vi "Target.vi"() -> ()   [LabVIEW 2017]
uses:
  shared/Kobuki Sensor Display.ctl
  controls/StatesEnum.ctl
  <vilib>/Platform/TimedLoop/XDataNode/timing_clust.ctl
  <vilib>/Platform/TimedLoop/XDataNode/nitl_modes.ctl
  <vilib>/Platform/TimedLoop/XDataNode/wakeup.ctl
  <vilib>/myRIO/Instrument Drivers/Onboard IO/UART/typedef/VISA Configuration.ctl
  shared/Sensors.ctl
  shared/Accelerometer.ctl
  Kobuki/KobukiSensors.ctl
  Kobuki/Kobuki Bumps and WheelDrops.ctl
  Kobuki/Kobuki Buttons.ctl
  <vilib>/myRIO/Common/Instrument Driver Framework/myRIO v1.0/UART/vis/myRIO v1.0 Close UART.vi
  <vilib>/myRIO/Common/Instrument Driver Framework/myRIO v1.0/myRIO v1.1 Open.vi
  Global Light Sensor.vi
  <vilib>/Instr/_visa.llb/VISA Configure Serial Port (Instr).vi
  <vilib>/myRIO/Common/Instrument Driver Framework/Utilities/vis/FPGA Ref Manager.vi
  <vilib>/myRIO/Common/Instrument Driver Framework/myRIO v1.0/myRIO v1.0 Reset FPGA.vi
  <vilib>/myRIO/Common/Instrument Driver Framework/myRIO v1.0/IRQ/vis/myRIO v1.0 IRQ Info FGV.vi
  <vilib>/myRIO/Common/Instrument Driver Framework/myRIO v1.0/IRQ/vis/myRIO v1.0 Timer IRQ Info FGV.vi
  <vilib>/myRIO/Common/Instrument Driver Framework/myRIO v1.0/IRQ/vis/myRIO v1.0 ISR Agent.vi
  <vilib>/Platform/TimedLoop/XDataNode/XDataNode.xnode
  <vilib>/myRIO/Express VI/Onboard IO/UART/UART Express VI.xnode
  <vilib>/myRIO/Instrument Drivers/Utilities/Utilities.lvlib
  <vilib>/Platform/TimedLoop/XDataNode/XDNodeRunTimeDep.lvlib
  <vilib>/myRIO/Instrument Drivers/Onboard IO/UART/UART.lvlib
panel:
  in  "Pause":bool
  in  "Tab Control":T1(tab)
  out "Kobuki Sensors (graphical)":T2 {"Right Wheel (mm/s)" scale=-500.0..500.0; "Left Wheel (mm/s)" scale=-500.0..500.0}
  out "Charge Status":i8(ring) items=["DISCHARGING"=0, "DOCKING_CHARGED"=2, "DOCKING_CHARGING"=6, "ADAPTER_CHARGED"=18, "ADAPTER_CHARGING"=22]
  out "Kobuki Battery Voltage":dbl(knob)=12000.0 scale=12.0..16.4 scale format="%#.1f"
  out "CurrentState":T4
  out "Loop Duration":i64
  out "error out":errorcluster
  in  "stop":bool
  out "Target Running":bool
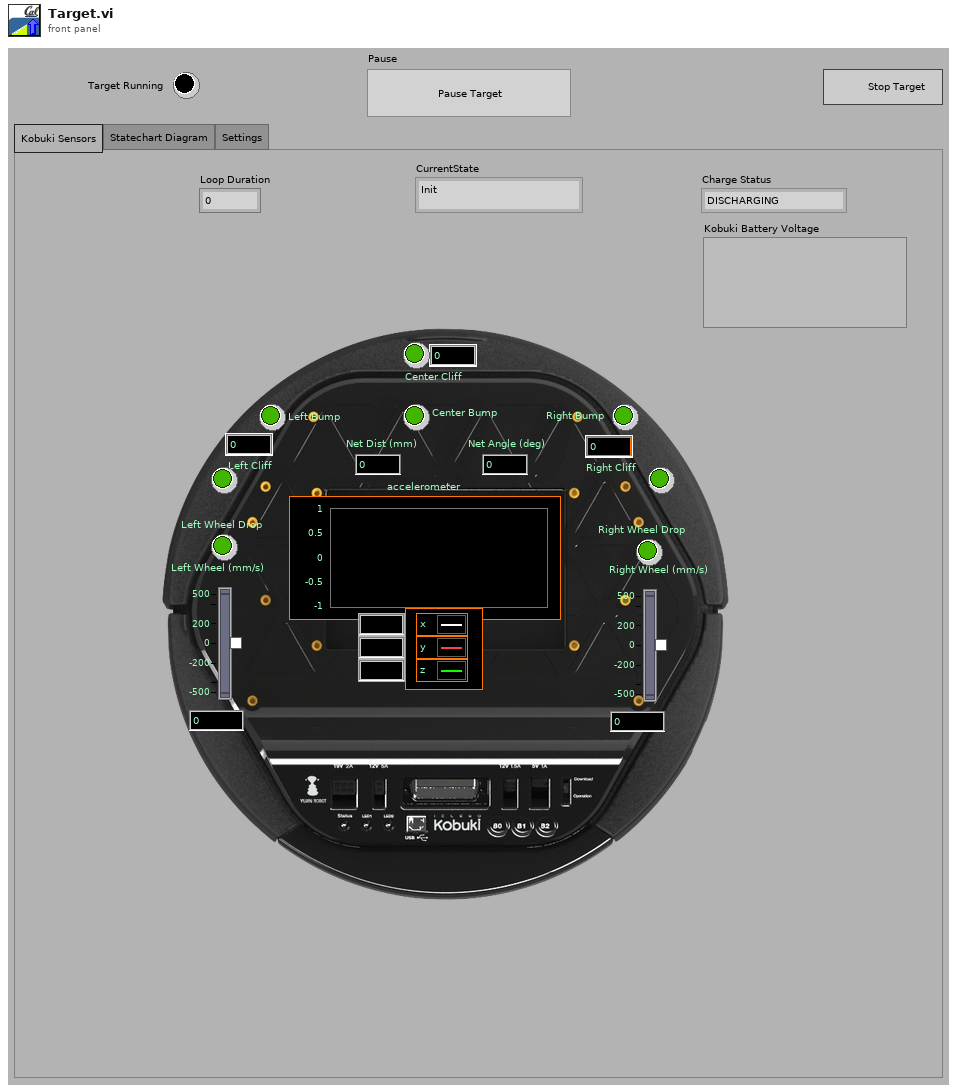
[diagram p1: front panel]
types:
  T1 = enum32{"Kobuki Sensors", "Statechart Diagram", "Settings"}
  T2 = typedef "Kobuki Sensor Display.ctl" = cluster{"Center Bump":bool, "Left Wheel Drop":bool, "Right Wheel Drop":bool, "Left Bump":bool, "Right Bump":bool, "Left Cliff":bool, "Center Cliff":bool, "Right Cliff":bool, "Net Dist (mm)":i32, "Net Angle (deg)":i32, "Left Cliff":u16, "Center Cliff":u16, "Right Cliff":u16, "  Left Wheel (mm/s)":i16, "Right Wheel (mm/s)":i16, "accelerometer":T3}
  T3 = typedef "Accelerometer.ctl" = cluster{"x axis (g)":dbl, "y axis (g)":dbl, "z axis (g)":dbl}
  T4 = typedef "StatesEnum.ctl" = enum16{"Init", "Center Cliff\n", "Pause", "Drive", "U.Turn", "L.Cliff", "R.Cliff", "Shut", "L.Bump", "R.Bump", "Red Light"}
  T5 = typedef "XDNodeRunTimeDep.lvlib/timing_clust.ctl" = cluster{"Expected End [f-1]":u64, "Actual End [f-1]":u64, "Finished Late? [f-1]":bool, "Expected End [i-1]":u64, "Actual End [i-1]":u64, "Finished Late? [i-1]":bool, "Expected Start [i]":u64, "Actual Start [i]":u64, "Expected Start [f]":u64, "Actual Start [f]":u64, "Source Name":string, "Structure Name":string, "Period":i64, "Deadline":i64, "Offset":i64, "Start":i64, "Priority":i32, "Timeout":i32, "Mode":T6, "Wakeup Reason":T7, "Error":errorcluster, "Source Type":string, "Secondary Source Type":string, "Global End Time":u64, "Global Start Time":u64, "Frame Duration":u64, "Iteration Duration":u64, "Assigned CPU":i32, "I/O Scan Engine Mode":u32}
  T6 = typedef "XDNodeRunTimeDep.lvlib/nitl_modes.ctl" = enum32{"No Change", "Process missed periods, maintain original phase", "Discard missed periods, maintain original phase", "Process missed periods, ignore original phase", "Discard missed periods, ignore original phase"}
  T7 = typedef "XDNodeRunTimeDep.lvlib/wakeup.ctl" = enum32{"Normal", "Aborted", "Asynchronous wakeup", "Timing source error", "Timed loop error", "Timeout"}
  T8 = typedef "Sensors.ctl" = cluster{"net distance (mm)":i32, "net angle (deg)":i32, "accelerometer":T3, "Is Simulator?":bool, "Kobuki Sensors":T9, "Requested Left Wheel Velocity(mm/s)":i32, "Requested Right Wheel Velocity(mm/s)":i32, "Green Light Sensed":bool, "Red Light Sensed":bool}
  T9 = typedef "KobukiSensors.ctl" = cluster{"Bumps + Wheel Drops":T10, "Cliff Left":bool, "Cliff Center":bool, "Cliff Right":bool, "Cliff Left Signal":u16, "Cliff Center Signal":u16, "Cliff Right Signal":u16, "Buttons":T11, "Left Wheel Encoder (ticks)":u16, "Right Wheel Encoder (ticks) ":u16, "Left  Wheel PWM":i8, "Right Wheel PWM":i8, "Left Wheel OverCurrent":bool, "Right Wheel OverCurrent ":bool, "Right Wheel Current (x10mA)":i16, "Left  Wheel Current  (x10mA)":i16, "TimeStamp":u16, "Battery Voltage":dbl, "Angle( of 100deg)":i16, "Angle Rate( of 100 deg/sec)":i16, "Charger Source ":i8}
  T10 = typedef "Kobuki Bumps and WheelDrops.ctl" = cluster{"Wheeldrop Left":bool, "Wheeldrop Right":bool, "Bump Left":bool, "Bump Center":bool, "Bump Right":bool}
  T11 = typedef "Kobuki Buttons.ctl" = cluster{"B0":bool, "B1":bool, "B2":bool}
  T12 = typedef "Outputs.ctl" = cluster{"Left Wheel Speed (mm/s)":i16, "Right Wheel Speed (mm/s)":i16}
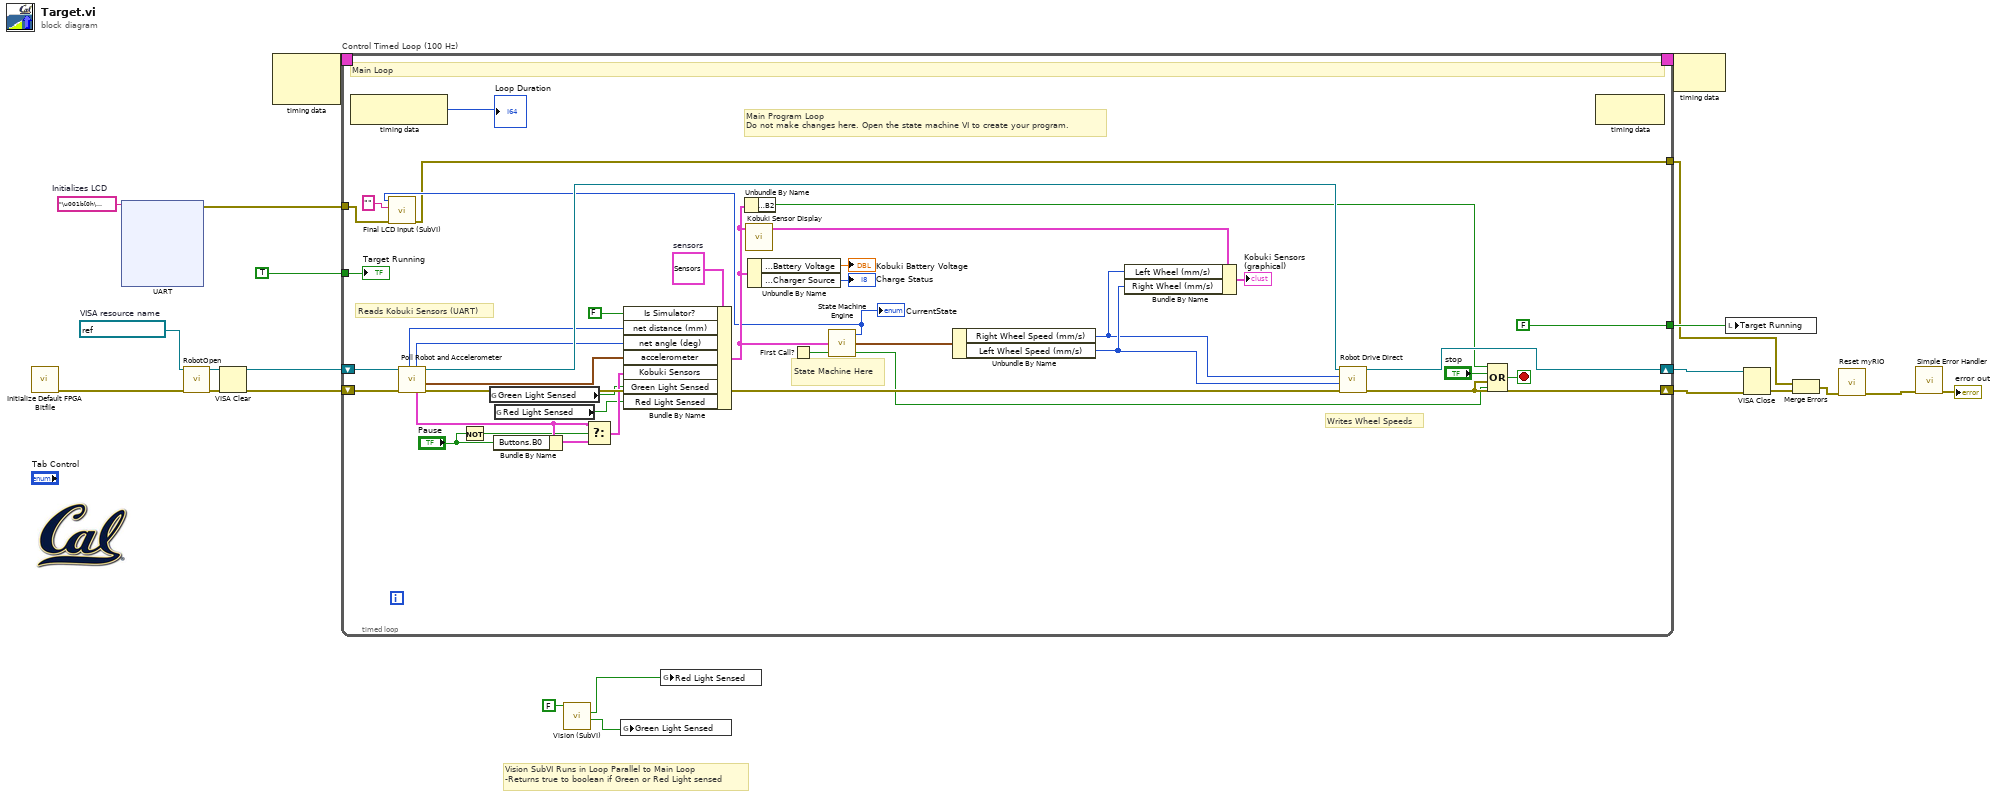
[diagram p0: block diagram]
diagram:
  w7 = "\u001b[0h\u001b[j"  # Initializes LCD
  w19 = refnum<visa-resource-name> "ASRL3::INSTR"  # VISA resource name
  # "Vision SubVI Runs in Loop Parallel to Main Loop\n-Returns true to boolean if Green or Red Light sensed"
  n1 = call <vilib>:"Initialize Default FPGA Bitfile.vi"() -> ("error out"=w17:errorcluster)  [unwired: 11 in]
  n2 = xnode "UART"("Characters to Write"=w7) -> ("error out"=w8:errorcluster)  [unwired: 1 in, 1 out]
  n3 = call "RobotOpen.vi"("error in (no error)"=w17, "Robot Communication port name"=w19) -> ("error out"=w15:errorcluster, "Robot Communication port name out"=w22:refnum<visa-resource-name>)  [unwired: 8 in]
  n4 = VISA Clear(VISA resource name=w22, error in (no error)=w15) -> (VISA resource name out=w13:refnum<visa-resource-name>, error out=w14:errorcluster)
  n5 = node-c288() -> (w10:T5)  [unwired: 2 in]
  n6 = timed-loop "Control Timed Loop (100 Hz)" {
    shift-right: [w60] -> w11
    shift-left: w13 -> [w57]
    shift-right: [w45] -> w12
    shift-left: w14 -> [w56]
    tunnel: TRUE ("stop") -> [w51]
    tunnel: [FALSE ("stop")] -> w20
    timing: w10 -> [_]
    timing-out: [_] -> w9
    tunnel: w8 -> [w28]
    tunnel: [w25] -> w5
    stop <- w59 stop-if-true
    w46 = T8 {"net distance (mm)"=0, "net angle (deg)"=0, "accelerometer"={"x axis (g)"=0.0, "y axis (g)"=0.0, "z axis (g)"=0.0}, "Is Simulator?"=FALSE, "Kobuki Sensors"={"Bumps + Wheel Drops"={"Wheeldrop Left"=FALSE, "Wheeldrop Right"=FALSE, "Bump Left"=FALSE, "Bump Center"=FALSE, "Bump Right"=FALSE}, "Cliff Left"=FALSE, "Cliff Center"=FALSE, "Cliff Right"=FALSE, "Cliff Left Signal"=0, "Cliff Center Signal"=0, "Cliff Right Signal"=0, "Buttons"={"B0"=FALSE, "B1"=FALSE, "B2"=FALSE}, "Left Wheel Encoder (ticks)"=0, "Right Wheel Encoder (ticks) "=0, "Left  Wheel PWM"=0, "Right Wheel PWM"=0, "Left Wheel OverCurrent"=FALSE, "Right Wheel OverCurrent "=FALSE, "Right Wheel Current (x10mA)"=0, "Left  Wheel Current  (x10mA)"=0, "TimeStamp"=0, "Battery Voltage"=0.0, "Angle( of 100deg)"=0, "Angle Rate( of 100 deg/sec)"=0, "Charger Source "=0}, "Requested Left Wheel Velocity(mm/s)"=0, "Requested Right Wheel Velocity(mm/s)"=0, "Green Light Sensed"=FALSE, "Red Light Sensed"=FALSE}  # sensors
    # "Main Program Loop\nDo not make changes here. Open the state machine VI to create your program."
    # "Writes Wheel Speeds"
    # "Reads Kobuki Sensors (UART)"
    # "State Machine Here"
    # "Main Loop"
    n7 = node-c288() -> (→"Loop Duration":i64)  [unwired: 1 in]
    n8 = call "Poll Robot and Accelerometer.vi"("error in"=w56, "UART in"=w57) -> ("error out"=w55:errorcluster, "Acceleration (g)"=w48:T3, "UART out"=w54:refnum<visa-resource-name>, "Kobuki Sensors  out"=w32:T9, "net angle (deg)"=w52:i32, "net distance (mm)"=w53:i32)  [unwired: 4 in]
    n9 = Not(x="Pause") -> (.not. x?=w29:bool)
    n10 = global read "Global Light Sensor.vi" "Green Light Sensed"() -> (w24:bool)
    n11 = Bundle By Name(cluster=w32, "Buttons.B0"="Pause") -> (w33:T9)
    n12 = global read "Global Light Sensor.vi" "Red Light Sensed"() -> (w23:bool)
    n13 = Select(t=w32, s=w29, f=w33) -> (s? t:f=w31:T9)
    n14 = Bundle By Name(cluster=w46, "Is Simulator?"=FALSE, "net distance (mm)"=w53, "net angle (deg)"=w52, "accelerometer"=w48, "Kobuki Sensors"=w31, "Green Light Sensed"=w24, "Red Light Sensed"=w23) -> (w38:T8)
    n15 = Unbundle By Name(w38) -> ("Kobuki Sensors.Buttons.B2"=w49:bool)
    n16 = call "Kobuki Sensor Display.vi"("sensors"=w38) -> ("Kobuki Sensors Display"=w35:T2)  [unwired: 4 in]
    n17 = Unbundle By Name(w38) -> ("Kobuki Sensors.Battery Voltage"=→"Kobuki Battery Voltage":dbl, "Kobuki Sensors.Charger Source"=→"Charge Status":i8)
    n18 = First Call?() -> (First Call?: T/F=w40:bool)
    n19 = call "State Machine Engine.vi"("Init?"=w40, "Inputs"=w38) -> ("Terminated?"=w39:bool, "Outputs"=w43:T12, "state out"=w26:T4)  [unwired: 1 in]
    "CurrentState" <- w26
    n20 = call "Final LCD Input (SubVI).vi"("error in (no error)"=w28, "String Input"="", "state input"=w26) -> ("error out"=w25:errorcluster)  [unwired: 8 in]
    n21 = Unbundle By Name(w43) -> ("Right Wheel Speed (mm/s)"=w36:i16, "Left Wheel Speed (mm/s)"=w37:i16)
    n22 = Bundle By Name(cluster=w35, "Left Wheel (mm/s)"=w36, "Right Wheel (mm/s)"=w37) -> (→"Kobuki Sensors (graphical)":T2)
    n23 = call "Robot Drive Direct.vi"("error in"=w55, "Left Wheel Velocity (mm/s)"=w37, "Right Wheel Velocity (mm/s)"=w36, "UART port in"=w54) -> ("error out"=w45:errorcluster, "UART port out"=w60:refnum<visa-resource-name>)  [unwired: 6 in]
    n24 = Compound Arithmetic op=OR(w49, "stop", w45, w39) -> (w59:bool)
    n25 = node-c288() -> ()  [unwired: 1 in, 1 out]
    "Target Running" <- w51
  }
  n26 = call "Vision (SubVI).vi"("stop"=FALSE) -> ("GREEN?"=w2:bool, "RED?"=w1:bool)  [unwired: 7 in, 2 out]
  n27 = global write "Global Light Sensor.vi" "Green Light Sensed"(w2) -> ()
  n28 = global write "Global Light Sensor.vi" "Red Light Sensed"(w1) -> ()
  n29 = node-c288(w9) -> ()  [unwired: 1 out]
  n30 = local write "Target Running"(w20) -> ()
  n31 = VISA Close(VISA resource name=w11, error in (no error)=w12) -> (error out=w6:errorcluster)
  n32 = Merge Errors(w5, w6) -> (w4:errorcluster)
  n33 = call <vilib>:"Reset myRIO.vi"("error in (no error)"=w4) -> ("error out"=w18:errorcluster)  [unwired: 10 in]
  n34 = call <vilib>:"Simple Error Handler.vi"("error in (no error)"=w18) -> ("error out"=→"error out":errorcluster)  [unwired: 4 in, 4 out]
